vi "GetReference.vi"(8 "error in":errorcluster, 11 "CaseStructure in":refnum<class "CaseStructure.lvclass">) -> (0 "error out":errorcluster, 1 "reference out":refnum<vi>, 3 "CaseStructure out":refnum<class "CaseStructure.lvclass">)   [LabVIEW 2014, in "CaseStructure.lvclass"]
uses:
  CaseStructure.lvclass
  Generic/Generic.lvclass
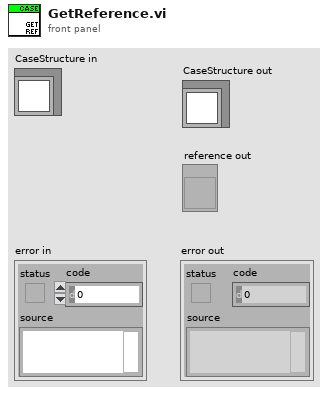
[diagram p1: front panel]
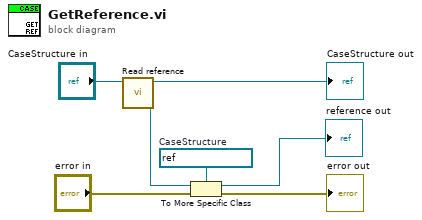
[diagram p0: block diagram]
diagram:
  w6 = refnum<vi> refnum  # CaseStructure
  n1 = call "Read reference.vi"("GObject in"="CaseStructure in") -> ("reference"=w5:refnum<vi>, "GObject out"=→"CaseStructure out":refnum<class "CaseStructure.lvclass">)  [unwired: 6 in, 1 out]
  n2 = To More Specific Class(target class=w6, reference=w5, error in="error in") -> (specific class reference=→"reference out":refnum<vi>, error out=→"error out":errorcluster)
